vi "path_constants.vi"() -> ()   [LabVIEW 2015]
uses:
  <vilib>/Utility/Data Type/NI_Data Type.lvlib
panel:
  out "Cluster Elements":variant[](array[variant])
  out "path 2":path
  out "path":path
  out "App:Default Data Directory":path
  out "Application Directory":path
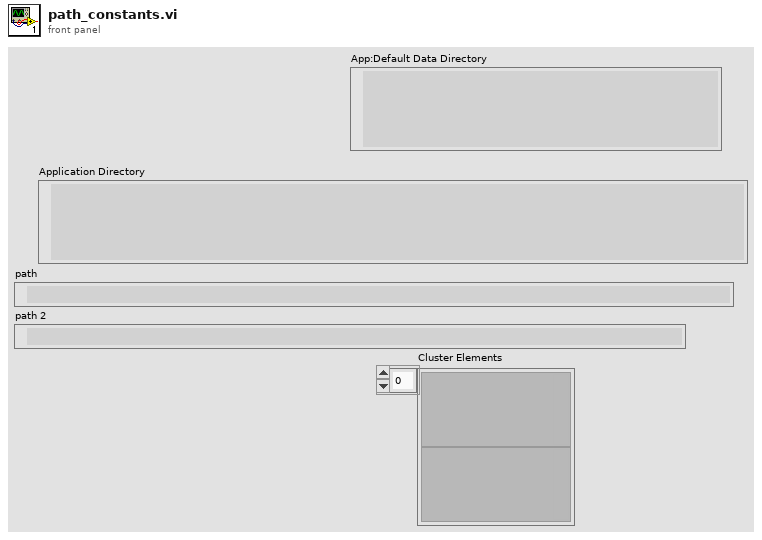
[diagram p1: front panel]
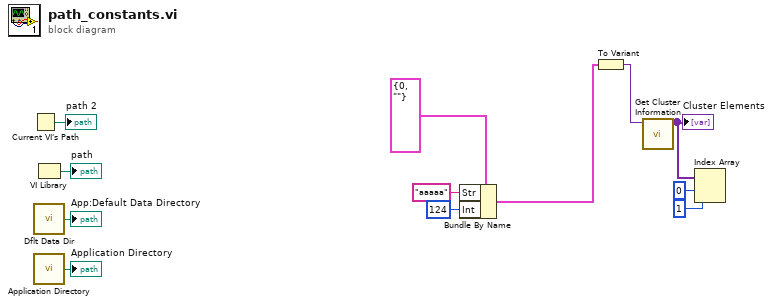
[diagram p0: block diagram]
diagram:
  n1 = Current VI's Path() -> (path=→"path 2":path)
  n2 = VI Library() -> (path=→"path":path)
  n3 = call <vilib>:"Dflt Data Dir.vi"() -> ("App:Default Data Directory"=→"App:Default Data Directory":path)
  n4 = call <vilib>:"Application Directory.vi"() -> ("Application Directory"=→"Application Directory":path)
  n5 = Bundle By Name(cluster=cluster{"Int":i32, "Str":string} {"Int"=0, "Str"=""} ("input cluster"), "Str"="aaaaa", "Int"=124) -> (w5:cluster{"Int":i32, "Str":string})
  n6 = To Variant(anything=w5) -> (Variant=w1:variant)
  n7 = call <vilib>:"Get Cluster Information.vi"("Variant"=w1) -> ("Cluster Elements"=w4:variant[])  [unwired: 9 in, 1 out]
  "Cluster Elements" <- w4
  n8 = Index Array(array=w4, index #1=0 ("index"), index #2=1 ("index")) -> ()  [unwired: 2 out]
